vi "forwardForInchMotionControl.vi"(9 "DistanceR (in)":dbl, 10 "DistanceL (in)":dbl, 11 "RobotDriveDevRef in":T1) -> (3 "RobotDriveDevRef out":T1)   [LabVIEW 2015]
uses:
  <vilib>/Rock Robotics/WPI/RobotDrive/WPI_RobotDriveDevRef.ctl
  <vilib>/Rock Robotics/WPI/MotorControl/WPI_MotorControlDeviceRef.ctl
  <vilib>/Rock Robotics/WPI/MotorControl/WPI_MotorControlType.ctl
  <vilib>/Rock Robotics/SystemInterfaces/DIO/FPGA_DIOPWMChannel.ctl
  <vilib>/Rock Robotics/WPI/PWM/WPI_PWMDeadband.ctl
  <vilib>/Rock Robotics/WPI/CAN/Jaguar/SubVIs/WPI_CANJaguar_ControlMode.ctl
  <vilib>/Rock Robotics/WPI/CAN/TalonSRX/WPI_CANTalonSRX_APIControlMode.ctl
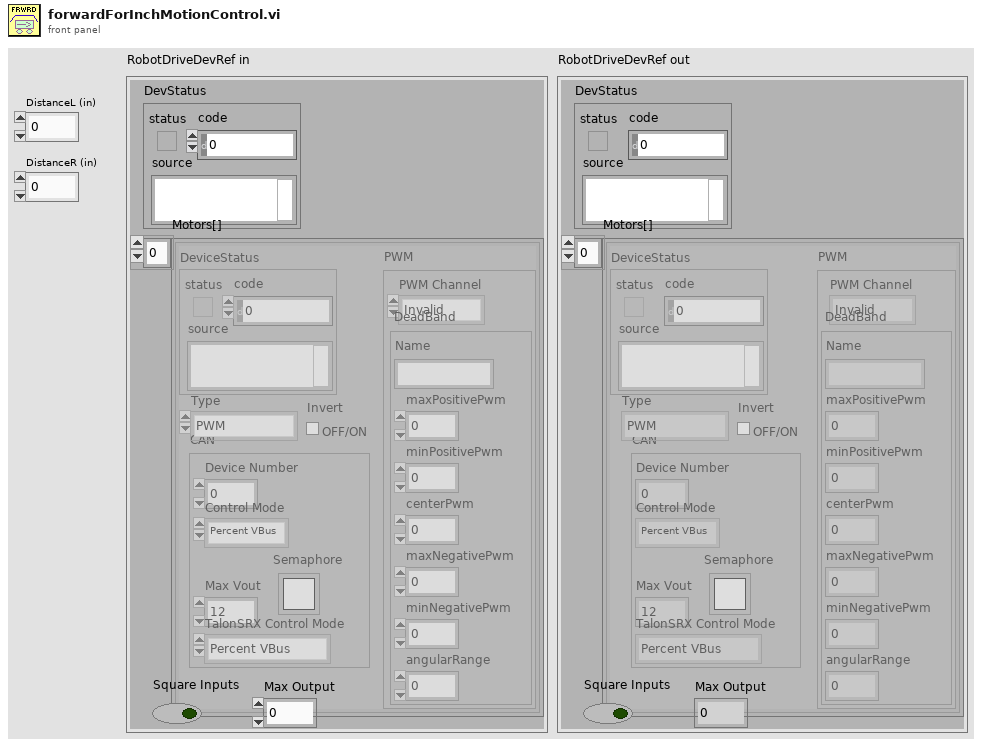
[diagram p1: front panel]
types:
  T1 = typedef "WPI_RobotDriveDevRef.ctl" = cluster{"DevStatus":errorcluster, "Motors[]":T2[], "Square Inputs":bool, "Max Output":dbl}
  T2 = typedef "WPI_MotorControlDeviceRef.ctl" = cluster{"DeviceStatus":errorcluster, "Type":T3, "PWM":cluster{"PWM Channel":T4, "DeadBand":T5}, "CAN":cluster{"Device Number":u8, "Control Mode":T6, "Semaphore":T7, "Max Vout":dbl, "TalonSRX Control Mode":T8}, "Invert":bool}
  T3 = typedef "WPI_MotorControlType.ctl" = enum16{"PWM", "CAN", "CANTalonSRX"}
  T4 = typedef "FPGA_DIOPWMChannel.ctl" = enum8{"PWM 0", "PWM 1", "PWM 2", "PWM 3", "PWM 4", "PWM 5", "PWM 6", "PWM 7", "PWM 8", "PWM 9", "PWM MXP 0", "PWM MXP 1", "PWM MXP 2", "PWM MXP 3", "PWM MXP 4", "PWM MXP 5", "PWM MXP 6", "PWM MXP 7", "PWM MXP 8", "PWM MXP 9", "Invalid"}
  T5 = typedef "WPI_PWMDeadband.ctl" = cluster{"Name":string, "maxPositivePwm":i32, "minPositivePwm":i32, "centerPwm":i32, "maxNegativePwm":i32, "minNegativePwm":i32, "angularRange":u16}
  T6 = typedef "WPI_CANJaguar_ControlMode.ctl" = enum8{"Percent VBus", "Current", "Speed", "Position", "Voltage"}
  T7 = typedef "Semaphore RefNum" = refnum<k1>
  T8 = typedef "WPI_CANTalonSRX_APIControlMode.ctl" = enum8{"Percent VBus", "Speed", "Position", "Slave", "Unchanged / Invalid", "Voltage Compensation", "Current", "Motion Profile"}
  T9 = typedef "WPI_PotentiometerDevRef.ctl" = cluster{"DevStatus":errorcluster, "Analog Channel":T10, "Invert Output":bool}
  T10 = typedef "FPGA_AIChannel.ctl" = enum8{"AI 0", "AI 1", "AI 2", "AI 3", "AI MXP 0", "AI MXP 1", "AI MXP 2", "AI MXP 3", "Invalid"}
  T11 = cluster{"Positions":dbl[], "Velocities":dbl[], "Accelerations":dbl[]}
  T12 = cluster{"kV":dbl, "kA":dbl, "PV":dbl, "PP":dbl, "DV":dbl}
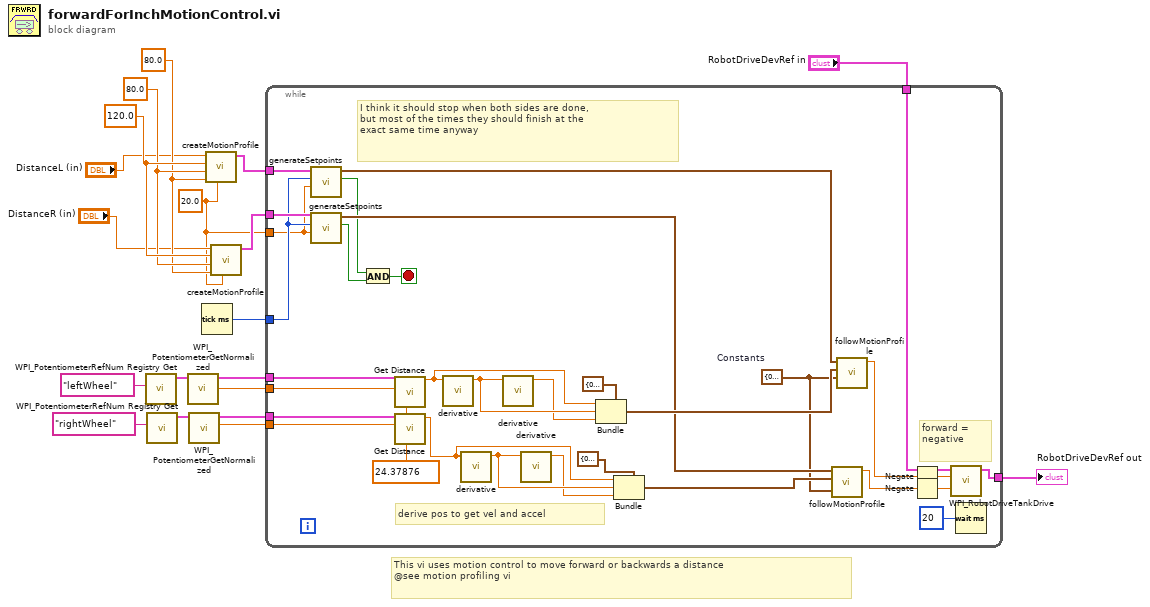
[diagram p0: block diagram]
diagram:
  w1 = 20.0 ("Motion Profile Control Frame Rate")
  w7 = 80.0 ("Max Acceleration (In/sec^2)")
  w8 = 80.0 ("Max Acceleration (In/sec^2)")
  w9 = 120.0 ("Max Speed (In/sec)")
  # "This vi uses motion control to move forward or backwards a distance\n@see motion profiling vi"
  n1 = call <vilib>:"WPI_PotentiometerRefNum Registry Get.vi"("refnum name"="leftWheel") -> ("PotDevRef"=w19:T9)  [unwired: 9 in, 1 out]
  n2 = call <vilib>:"WPI_PotentiometerRefNum Registry Get.vi"("refnum name"="rightWheel") -> ("PotDevRef"=w18:T9)  [unwired: 9 in, 1 out]
  n3 = call <vilib>:"WPI_PotentiometerGetNormalized.vi"("PotDevRef"=w19) -> ("Normalized Value"=w14:dbl, "PotDevRef"=w15:T9)  [unwired: 8 in, 1 out]
  n4 = call <vilib>:"WPI_PotentiometerGetNormalized.vi"("PotDevRef"=w18) -> ("Normalized Value"=w12:dbl, "PotDevRef"=w13:T9)  [unwired: 8 in, 1 out]
  n5 = Tick Count (ms)() -> (millisecond timer value=w2:u32)
  n6 = call "createMotionProfile.vi"("ms per frame"=w1, "Max Jerk (In/sec^3)"=w7, "Max Acceleration (In/sec^2)"=w8, "Max Speed (In/sec)"=w9, "Inches to Travel"="DistanceL (in)") -> ("Profile"=w4:T11)  [unwired: 6 in]
  n7 = call "createMotionProfile.vi"("ms per frame"=w1, "Max Jerk (In/sec^3)"=w7, "Max Acceleration (In/sec^2)"=w8, "Max Speed (In/sec)"=w9, "Inches to Travel"="DistanceR (in)") -> ("Profile"=w3:T11)  [unwired: 6 in]
  n8 = while {
    tunnel: w4 -> [w48]
    tunnel: w3 -> [w43]
    tunnel: w15 -> [w36]
    tunnel: w14 -> [w35]
    tunnel: w13 -> [w34]
    tunnel: w12 -> [w33]
    tunnel: "RobotDriveDevRef in" -> [w32]
    tunnel: [w31] -> w11
    tunnel: w2 -> [w25]
    tunnel: w1 -> [w24]
    stop <- w37 stop-if-true
    w40 = T12 {"kV"=0.0086, "kA"=0.0004, "PV"=0.02, "PP"=0.5, "DV"=0.0}  # Constants
    w50 = 24.37876 ("distance/rotation")
    # "forward =\nnegative"
    # "I think it should stop when both sides are done, \nbut most of the times they should finish at the\nexact same time anyway"
    # "derive pos to get vel and accel"
    n9 = call "generateSetpoints.vi"("ms/frame"=w24, "start time"=w25, "Profile"=w48) -> ("Done?"=w39:bool, "Setpoint"=w45:cluster{"pos":dbl, "vel":dbl, "accel":dbl})  [unwired: 7 in]
    n10 = call "generateSetpoints.vi"("ms/frame"=w24, "start time"=w25, "Profile"=w43) -> ("Done?"=w38:bool, "Setpoint"=w42:cluster{"pos":dbl, "vel":dbl, "accel":dbl})  [unwired: 7 in]
    n11 = And(x=w39, y=w38) -> (x .and. y?=w37:bool)
    n12 = call "Get Distance.vi"("distance/rotation"=w50, "Starting value"=w35, "PotDevRef"=w36) -> ("Distance"=w26:dbl)  [unwired: 8 in]
    n13 = call "Get Distance.vi"("distance/rotation"=w50, "Starting value"=w33, "PotDevRef"=w34) -> ("Distance"=w28:dbl)  [unwired: 8 in]
    n14 = call "derivative.vi"("x"=w26) -> ("dx/dt"=w47:dbl)  [unwired: 10 in]
    n15 = call "derivative.vi"("x"=w28) -> ("dx/dt"=w46:dbl)  [unwired: 10 in]
    n16 = call "derivative.vi"("x"=w47) -> ("dx/dt"=w27:dbl)  [unwired: 10 in]
    n17 = call "derivative.vi"("x"=w46) -> ("dx/dt"=w29:dbl)  [unwired: 10 in]
    n18 = Bundle(cluster=cluster{"pos":dbl, "vel":dbl, "accel":dbl} {"pos"=0.0, "vel"=0.0, "accel"=0.0}, "pos"=w26, "vel"=w47, "accel"=w27) -> (w44:cluster{"pos":dbl, "vel":dbl, "accel":dbl})
    n19 = Bundle(cluster=cluster{"pos":dbl, "vel":dbl, "accel":dbl} {"pos"=0.0, "vel"=0.0, "accel"=0.0}, "pos"=w28, "vel"=w46, "accel"=w29) -> (w41:cluster{"pos":dbl, "vel":dbl, "accel":dbl})
    n20 = call "followMotionProfile.vi"("Constants"=w40, "Feedback"=w41, "Target"=w42) -> ("Duty Cycle"=w22:dbl)  [unwired: 8 in]
    n21 = call "followMotionProfile.vi"("Constants"=w40, "Feedback"=w44, "Target"=w45) -> ("Duty Cycle"=w20:dbl)  [unwired: 8 in]
    n22 = Negate(x=w20) -> (-x=w21:dbl)
    n23 = Negate(x=w22) -> (-x=w23:dbl)
    n24 = call <vilib>:"WPI_RobotDriveTankDrive.vi"("Right axis value"=w23, "Left axis value"=w21, "RobotDriveDevRef"=w32) -> ("RobotDriveDevRef"=w31:T1)  [unwired: 6 in, 2 out]
    n25 = Wait (ms)(milliseconds to wait=u32 20) -> ()  [unwired: 1 out]
  }
  "RobotDriveDevRef out" <- w11
